vi "Unpack Control Key Down.vi"(0 "ControlKeyDownMsg":refnum<class "ControlKeyDownMsg.lvclass">) -> (2 "FocusObj":refnum<vi>, 3 "ScanCode":i16, 4 "CtlRef":refnum<vi>, 6 "Control Label":string, 8 "Time":u32, 10 "Char":i16, 13 "PlatMods":T1, 14 "Mods":cluster{"Double Click":bool, "Menu Key":bool}, 15 "VKey":T2)   [LabVIEW 2020, in "MVA Framework.lvlib" / "ActorEvents.lvlib" / "ControlKeyDownMsg.lvclass"]
doc: "<License>\nCopyright © 2017 Composed Systems, LLC | All rights reserved\nwww.composed.io\n\nAuthor: Ethan Stern <ethan.stern@composed.io>\n\nThis software is provided \"AS IS\" WITHOUT WARRANTIES, either express or implied, AND IS FOR EDUCATIONAL PURPOSES ONLY.\n</License>"
uses:
  ControlKeyDownMsg.lvclass
  <vilib>/event_ctls.llb/eventvkey.ctl
  ControlKeyDownMsg.lvclass/ControlKeyDownMsg.ctl
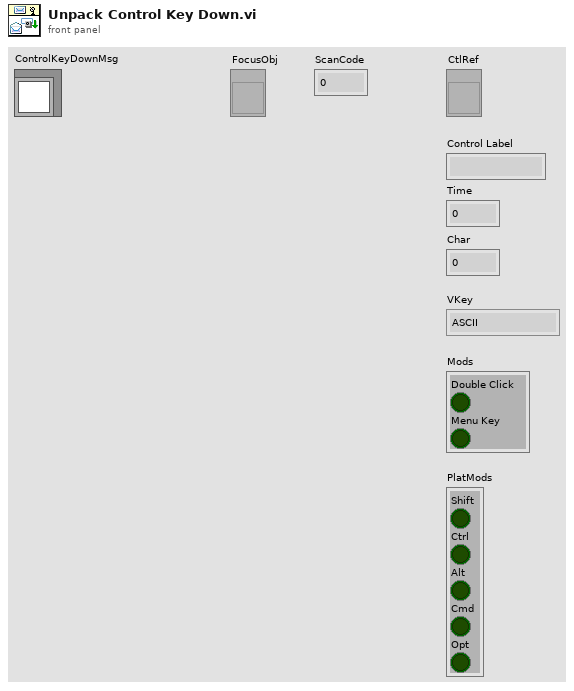
[diagram p1: front panel]
types:
  T1 = cluster{"Shift":bool, "Ctrl":bool, "Alt":bool, "Cmd":bool, "Opt":bool}
  T2 = typedef "eventvkey.ctl" = enum16{"ASCII", "Enter", "Return", "Shift", "Ctrl", "Alt", "Cmd", "Opt", "Caps", "NumLock", "Clear", "Break", "Up", "Down", "Left", "Right", "Insert", "Delete", "Home", "End", "PageUp", "PageDown", "Escape", "Help", "Pause", "ScrollLock", "F1", "F2", "F3", "F4", "F5", "F6", "F7", "F8", "F9", "F10", "F11", "F12", "F13", "F14", "F15", "F16", "F17", "F18", "F19", "F20", "F21", "F22", "F23", "F24", "Play", "VolumeUp", "VolumeDown", "Mute", "Two Byte Char"}
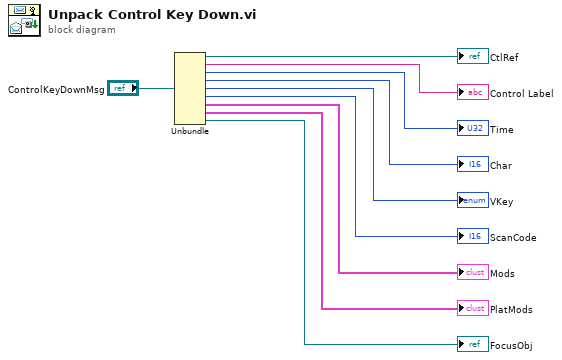
[diagram p0: block diagram]
diagram:
  n1 = Unbundle("ControlKeyDownMsg") -> (→"CtlRef":refnum<vi>, →"Control Label":string, →"Time":u32, →"Char":i16, →"VKey":T2, →"ScanCode":i16, →"Mods":cluster{"Double Click":bool, "Menu Key":bool}, →"PlatMods":T1, →"FocusObj":refnum<vi>)
